vi "ABAPI Dist Delay with Error.vi"(8 "error in (no error)":errorcluster, 9 "skip wait":bool, 10 "milliseconds to wait":u32=100) -> (0 "error out":errorcluster)   [LabVIEW 2020]
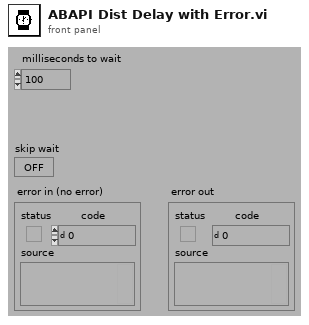
[diagram p1: front panel]
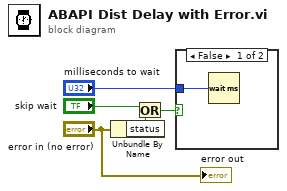
[diagram p0: block diagram]
diagram:
  n1 = Unbundle By Name("error in (no error)") -> ("status"=w3:bool)
  n2 = Or(x="skip wait", y=w3) -> (x .or. y?=w2:bool)
  n3 = case shown="False" w2 {
    tunnel: "milliseconds to wait" -> [w6 _]
    frame False {
      n4 = Wait (ms)(milliseconds to wait=w6) -> ()  [unwired: 1 out]
    }
    frame True {
    }
  }
  "error out" <- "error in (no error)"
